vi "VS_Function_versionX.vi"() -> (3 "VeriStand version info":T1={"VeriStand.exe Path"="", "Assembly"="", "Constructor Token"=0, "Module Token"={"GetIWorkspaceToken"=100663761, "GetIStimulusToken"=100663772, "GetIModelManagerToken"=100663768, "GetIProjectToken"=100663780, "RunProjectToken"=100663643, "CloseProjectToken"=100663640, "RunWorkspaceToken"=100663694, "StopWorkspaceToken"=100663695, "SetSingleChannelToken"=100663609, "SetMultipleParametersToken"=100663608, "RunStimulusToken"=100663670, "GetStimulusStateToken"=100663669, "Open WorkspaceToken"=0, "DeployToken"=0, "UndeployToken"=0, "QuitToken"=0}})   [LabVIEW 2011]
doc: "This VI is used to select the NI VeriStand dotNet Assembly version"
uses:
  SeqBuilder/Ctls/dotNetAssemblyInfo.ctl
  SeqBuilder/Ctls/VSModuleTokens.ctl
  <vilib>/Utility/sysdir.llb/System Directory Type.ctl
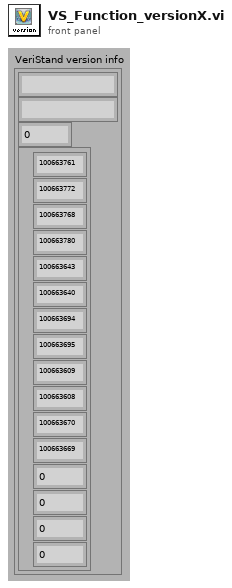
[diagram p1: front panel]
types:
  T1 = typedef "dotNetAssemblyInfo.ctl" = cluster{"VeriStand.exe Path":string, "Assembly":string, "Constructor Token":i32, "Module Token":T2}
  T2 = typedef "VSModuleTokens.ctl" = cluster{"GetIWorkspaceToken":i32, "GetIStimulusToken":i32, "GetIModelManagerToken":i32, "GetIProjectToken":i32, "RunProjectToken":i32, "CloseProjectToken":i32, "RunWorkspaceToken":i32, "StopWorkspaceToken":i32, "SetSingleChannelToken":i32, "SetMultipleParametersToken":i32, "RunStimulusToken":i32, "GetStimulusStateToken":i32, "Open WorkspaceToken":i32, "DeployToken":i32, "UndeployToken":i32, "QuitToken":i32}
  T3 = typedef "System Directory Type.ctl" = i32
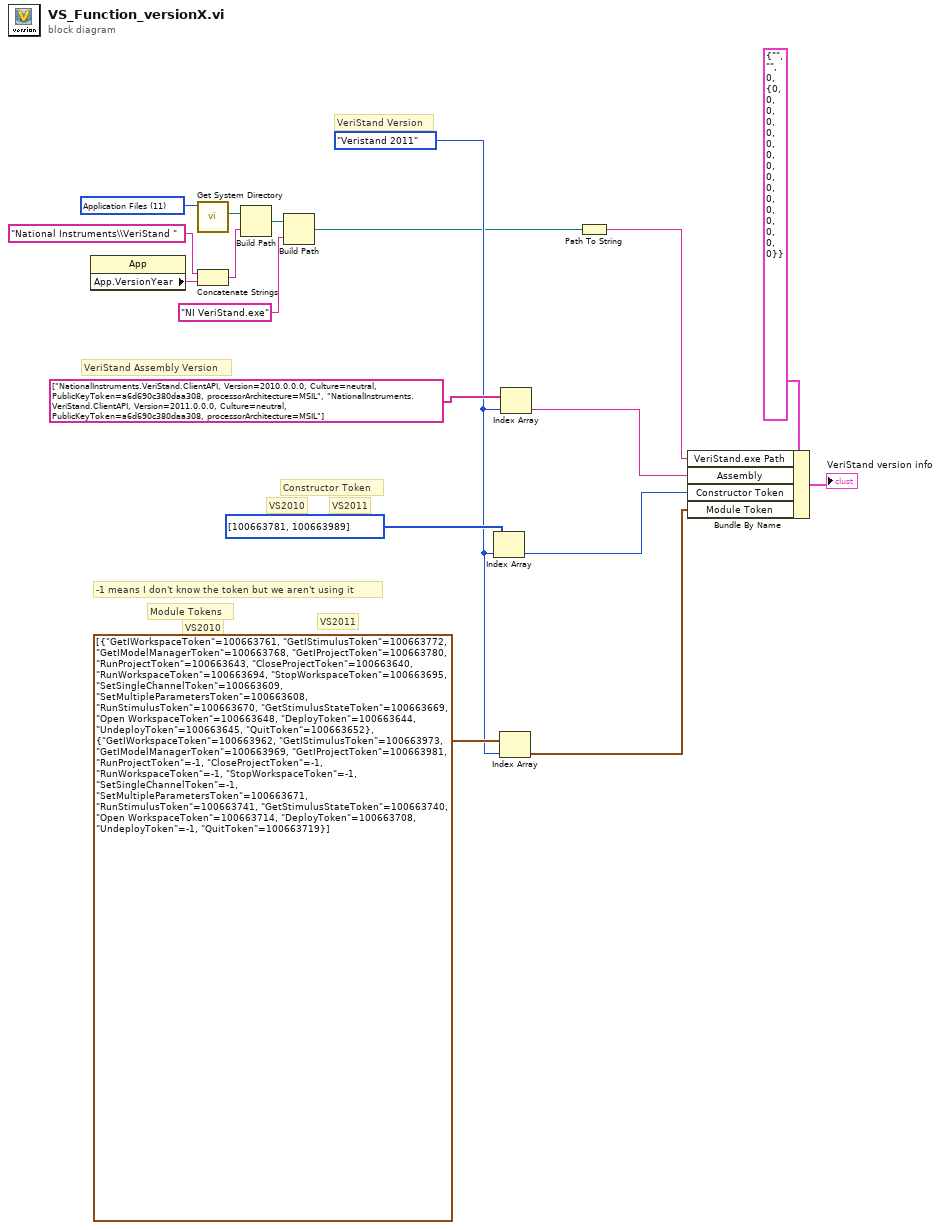
[diagram p0: block diagram]
diagram:
  w9 = T3 11 items=["User Home"=0, "User Desktop"=1, "User Documents"=2, "User Application Data"=3, "User Preferences"=4, "User Temporary"=5, "Public Documents"=6, "Public Application Data"=7, "Public Preferences"=8, "Public Cache"=13, "System Core Libraries"=9, "System Installed Libraries"=10, "Application Files"=11, "Boot Volume Root"=12] ("system directory type")
  w10 = enum16{"VeriStand 2010", "Veristand 2011"}."Veristand 2011"
  # "-1 means I don't know the token but we aren't using it"
  # "VS2011"
  # "VS2010"
  # "Module Tokens"
  # "VeriStand Version"
  # "VS2011"
  # "VS2010"
  # "Constructor Token"
  # "VeriStand Assembly Version"
  n1 = property class="App"() -> ("App.VersionYear"=w4:string)  [unwired: 2 in, 2 out]
  n2 = call <vilib>:"Get System Directory.vi"("system directory type"=w9) -> ("system directory"=w6:path)  [unwired: 10 in]
  n3 = Concatenate Strings("National Instruments\\VeriStand ", w4) -> (w3:string)
  n4 = Build Path(base path=w6, name or relative path=w3) -> (appended path=w8:path)
  n5 = Build Path(base path=w8, name or relative path="NI VeriStand.exe") -> (appended path=w2:path)
  n6 = Index Array(array=i32[] [100663781, 100663989], index=w10) -> (element=w13:i32)
  n7 = Index Array(array=T2[] [{"GetIWorkspaceToken"=100663761, "GetIStimulusToken"=100663772, "GetIModelManagerToken"=100663768, "GetIProjectToken"=100663780, "RunProjectToken"=100663643, "CloseProjectToken"=100663640, "RunWorkspaceToken"=100663694, "StopWorkspaceToken"=100663695, "SetSingleChannelToken"=100663609, "SetMultipleParametersToken"=100663608, "RunStimulusToken"=100663670, "GetStimulusStateToken"=100663669, "Open WorkspaceToken"=100663648, "DeployToken"=100663644, "UndeployToken"=100663645, "QuitToken"=100663652}, {"GetIWorkspaceToken"=100663962, "GetIStimulusToken"=100663973, "GetIModelManagerToken"=100663969, "GetIProjectToken"=100663981, "RunProjectToken"=-1, "CloseProjectToken"=-1, "RunWorkspaceToken"=-1, "StopWorkspaceToken"=-1, "SetSingleChannelToken"=-1, "SetMultipleParametersToken"=100663671, "RunStimulusToken"=100663741, "GetStimulusStateToken"=100663740, "Open WorkspaceToken"=100663714, "DeployToken"=100663708, "UndeployToken"=-1, "QuitToken"=100663719}], index=w10) -> (element=w11:T2)
  n8 = Index Array(array=string[] ["NationalInstruments.VeriStand.ClientAPI, Version=2010.0.0.0, Culture=neutral, PublicKeyToken=a6d690c380daa308, processorArchitecture=MSIL", "NationalInstruments.VeriStand.ClientAPI, Version=2011.0.0.0, Culture=neutral, PublicKeyToken=a6d690c380daa308, processorArchitecture=MSIL"] ("Assembly version"), index=w10) -> (element=w12:string)
  n9 = Path To String(path=w2) -> (string=w1:string)
  n10 = Bundle By Name(cluster=T1 {"VeriStand.exe Path"="", "Assembly"="", "Constructor Token"=0, "Module Token"={"GetIWorkspaceToken"=0, "GetIStimulusToken"=0, "GetIModelManagerToken"=0, "GetIProjectToken"=0, "RunProjectToken"=0, "CloseProjectToken"=0, "RunWorkspaceToken"=0, "StopWorkspaceToken"=0, "SetSingleChannelToken"=0, "SetMultipleParametersToken"=0, "RunStimulusToken"=0, "GetStimulusStateToken"=0, "Open WorkspaceToken"=0, "DeployToken"=0, "UndeployToken"=0, "QuitToken"=0}} ("dotNet Assembly Info 2"), "VeriStand.exe Path"=w1, "Assembly"=w12, "Constructor Token"=w13, "Module Token"=w11) -> (→"VeriStand version info":T1)
